vi "Check for VIM Extention.vi"(11 "VI Name in":string) -> (2 "Is a Malleable VI":bool, 3 "VI Name out":string)   [LabVIEW 2020, in "Peek Window.lvlib"]
uses:
  Peek Window.lvlib
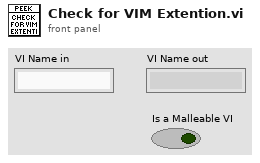
[diagram p1: front panel]
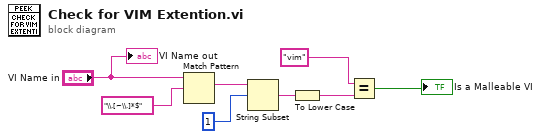
[diagram p0: block diagram]
diagram:
  n1 = Match Pattern(string="VI Name in", regular expression="\\.[~\\.]*$") -> (match substring=w3:string)  [unwired: 1 in, 3 out]
  n2 = String Subset(string=w3, offset (0)=1) -> (substring=w5:string)  [unwired: 1 in]
  n3 = To Lower Case(string=w5) -> (all lower case string=w6:string)
  n4 = Equal?(x="vim", y=w6) -> (x = y?=→"Is a Malleable VI":bool)
  "VI Name out" <- "VI Name in"
